vi "显示数据.vi"(8 "error in (no error)":errorcluster caption="错误输入（无错误）", 11 "数据分析 输入":refnum<class "数据分析.lvclass"> caption="DNL_LabVIEW Object in") -> (0 "error out":errorcluster caption="错误输出", 2 "采集数据":dbl[](array[numeric]), 3 "数据分析 输出":refnum<class "数据分析.lvclass"> caption="DNL_LabVIEW Object out")   [LabVIEW 2013, in "数据分析.lvclass"]
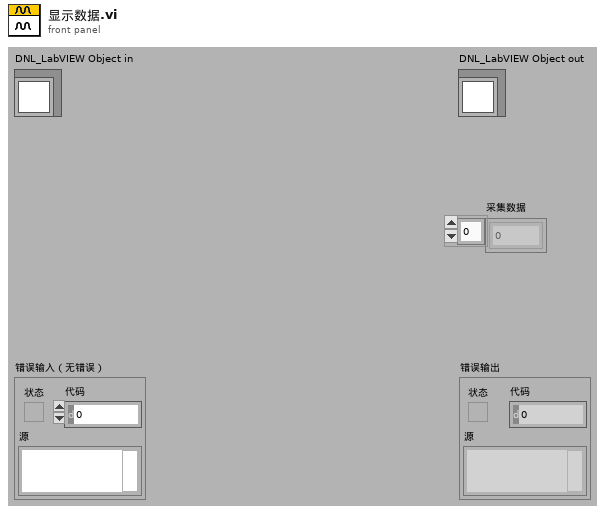
[diagram p1: front panel]
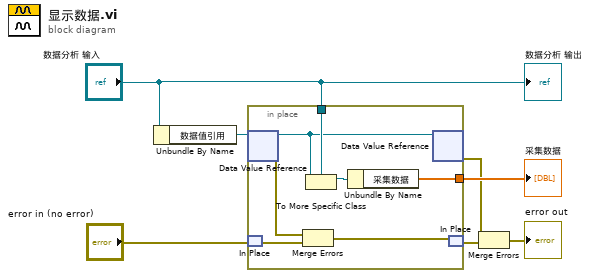
[diagram p0: block diagram]
diagram:
  n1 = Unbundle By Name("数据分析 输入") -> ("数据值引用"=w7:refnum<data-value>)
  n2 = in-place {
    in-place-border: "数据分析 输入" -> [w14]
    in-place-border: [w11] -> w5
    n3 = in-place-dvr #1(w7) -> (w13:refnum<class "订阅者接口.lvclass">, w9:errorcluster)
    n4 = in-place-match #2("error in (no error)") -> (w10:errorcluster)
    n5 = Merge Errors(w9, w10) -> (w8:errorcluster)
    n6 = To More Specific Class(target class=w14, reference=w13) -> (specific class reference=w12:refnum<class "数据分析.lvclass">)  [unwired: 1 in, 1 out]
    n7 = Unbundle By Name(w12) -> ("采集数据"=w11:dbl[])
    n8 = in-place-dvr #1(w13) -> (w2:errorcluster)  [unwired: 1 out]
    n9 = in-place-match #2(w8) -> (w3:errorcluster)
  }
  "采集数据" <- w5
  n10 = Merge Errors(w2, w3) -> (→"error out":errorcluster)
  "数据分析 输出" <- "数据分析 输入"
